vi "Edit PID.vi"(8 "error in (no error)":errorcluster, 11 "Node Ptr":u64 format="%.0x") -> (0 "error out":errorcluster)   [LabVIEW 2015, in "Diagnostics Addon System Explorer.lvlib"]
uses:
  Diagnostics Addon System Explorer.lvlib
  Shared/FG Action.ctl
  Shared/Get Signals from DIDPID.vi
  Shared/Signal Parameters FG.vi
  Shared/GUID Lookup.vi
  <vilib>/NI Veristand/Custom Device API/NI VeriStand - Set Item Property.vi
  <vilib>/NI Veristand/Custom Device API/Set Item Property (U32).vi
  <vilib>/NI Veristand/Custom Device API/NI VeriStand - Get Item Property.vi
  <vilib>/NI Veristand/Custom Device API/Get Item Property (U32).vi
  <vilib>/NI Veristand/Custom Device API/Set Item Property (Double).vi
  <vilib>/NI Veristand/Custom Device API/Set Item Property (String).vi
  <vilib>/NI Veristand/Custom Device API/Get Item Property (Double).vi
  <vilib>/NI Veristand/Custom Device API/Get Item Property (String).vi
  <vilib>/NI Veristand/Custom Device API/NI VeriStand - Get Item Description.vi
  <vilib>/NI Veristand/Custom Device API/NI VeriStand - Get Custom Device Channel Data.vi
  <vilib>/NI Veristand/Custom Device API/Custom Device API.lvlib
  Shared/Diagnostics Addon Shared.lvlib
  <vilib>/NI Veristand/Custom Device Tools/Custom Device Utility Library/Custom Device Utility Library.lvlib
panel:
  in  "Tag":string
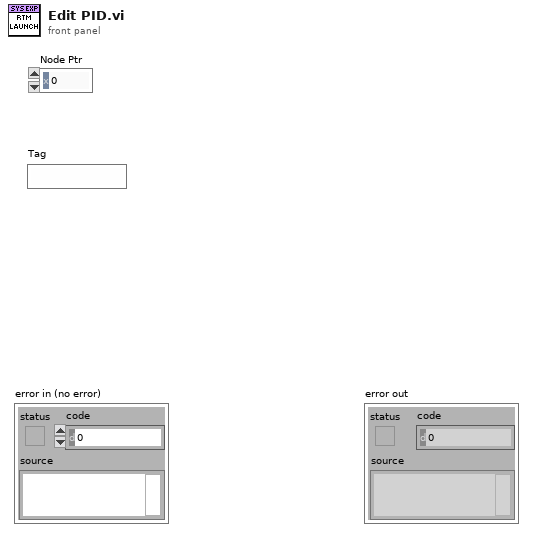
[diagram p1: front panel]
types:
  T1 = typedef "Diagnostics Addon Shared.lvlib/DIDPID Parameters.ctl" = cluster{"Name":string, "Description":string, "ID":u16, "Signals":T2[]}
  T2 = typedef "Diagnostics Addon Shared.lvlib/DIDPID Signal Parameters.ctl" = cluster{"Start Bit":u8, "Length":u8, "Scaling Factor":dbl, "Scaling Offset":dbl, "Minimum":dbl, "Maximum":dbl, "Data Type":u32, "Byte Order":u32, "Default Value":dbl, "Name":string, "Units":string, "Description":string}
  T3 = typedef "Custom Device API.lvlib/Custom Device Item Ref.ctl" = u64
  T4 = typedef "Custom Device API.lvlib/Custom Device Item Info.ctl" = cluster{"Name":string, "Is Channel":bool, "GUID":string, "Is Waveform":bool}
  T5 = typedef "Diagnostics Addon Shared.lvlib/FG Action.ctl" = enum16{"Get", "Set"}
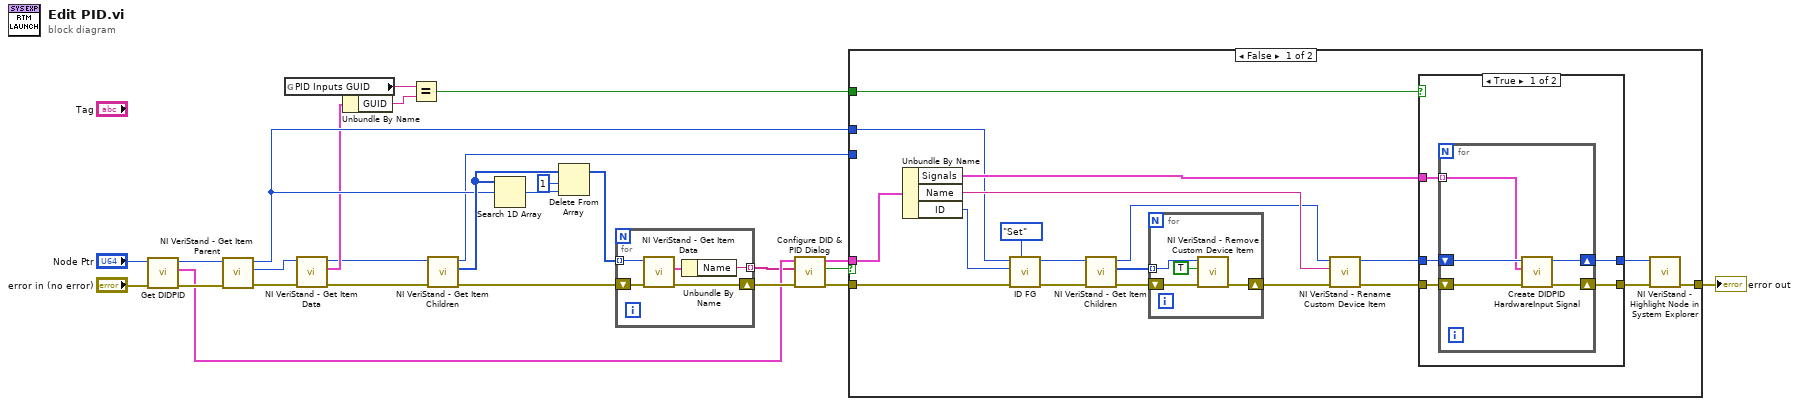
[diagram p0: block diagram]
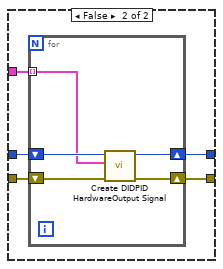
[diagram p2: hidden frame]
diagram:
  n1 = call "Get DIDPID.vi"("error in (no error)"="error in (no error)", "Item Ref in"="Node Ptr") -> ("error out"=w16:errorcluster, "PID In"=w13:T1, "Item Ref out"=w14:T3)  [unwired: 7 in]
  n2 = call <vilib>:"NI VeriStand - Get Item Parent.vi"("error in (no error)"=w16, "Item Ref in"=w14) -> ("error out"=w5:errorcluster, "Parent Ref"=w4:T3, "Item Ref out"=w11:T3)  [unwired: 6 in, 1 out]
  n3 = global read "GUID Lookup.vi" "PID Inputs GUID"() -> (w7:string)
  n4 = call <vilib>:"NI VeriStand - Get Item Data.vi"("error in (no error)"=w5, "Item Ref in"=w4) -> ("error out"=w2:errorcluster, "Item Info"=w8:T4, "Item Ref out"=w3:T3)  [unwired: 6 in, 1 out]
  n5 = Unbundle By Name(w8) -> ("GUID"=w6:string)
  n6 = Equal?(x=w7, y=w6) -> (x = y?=w1:bool)
  n7 = call <vilib>:"NI VeriStand - Get Item Children.vi"("error in (no error)"=w2, "Item Ref in"=w3) -> ("error out"=w26:errorcluster, "Child Refs"=w25:T3[], "Item Ref out"=w10:T3)  [unwired: 6 in, 1 out]
  n8 = Search 1D Array(1D array=w25, element=w11) -> (index of element=w23:i32)  [unwired: 1 in]
  n9 = Delete From Array(array=w25, length=1, index=w23) -> (array with subset deleted=w24:T3[])  [unwired: 1 out]
  n10 = for {
    tunnel: [w29] -> w12 mode=indexing
    shift-right: [w28] -> w18
    shift-left: w26 -> [w30]
    tunnel: w24 -> [w27] mode=indexing
    n11 = call <vilib>:"NI VeriStand - Get Item Data.vi"("error in (no error)"=w30, "Item Ref in"=w27) -> ("error out"=w28:errorcluster, "Item Info"=w31:T4)  [unwired: 8 out]
    n12 = Unbundle By Name(w31) -> ("Name"=w29:string)
  }
  n13 = call "Configure DID & PID Dialog.vi"("error in (no error)"=w18, "Existing PIDs"=w12, "Parameters In"=w13) -> ("error out"=w20:errorcluster, "Cancel PID?"=w19:bool, "Parameters Out"=w21:T1)  [unwired: 6 in]
  n14 = case shown="False" w19 {
    tunnel: w20 -> [w33 w75]
    tunnel: w10 -> [_ _]
    tunnel: w21 -> [w50 _]
    tunnel: [w44 w75] -> w9
    tunnel: w11 -> [w36 _]
    tunnel: w1 -> [w38 _]
    frame False {
      n15 = Unbundle By Name(w50) -> ("Signals"=w41:T2[], "Name"=w49:string, "ID"=w32:u16)
      n16 = call "ID FG.vi"("Action"=FG_Action."Set", "error in (no error)"=w33, "ID"=w32, "Device Item Ref in"=w36) -> ("error out"=w34:errorcluster, "Device Item Ref out"=w35:T3)  [unwired: 5 in, 1 out]
      n17 = call <vilib>:"NI VeriStand - Get Item Children.vi"("error in (no error)"=w34, "Item Ref in"=w35) -> ("error out"=w47:errorcluster, "Child Refs"=w48:T3[], "Item Ref out"=w45:T3)  [unwired: 6 in, 1 out]
      n18 = for {
        tunnel: w48 -> [w74] mode=indexing
        shift-right: [w71] -> w46
        shift-left: w47 -> [w73]
        n19 = call <vilib>:"NI VeriStand - Remove Custom Device Item.vi"("error in (no error)"=w73, "Force Delete (F)"=TRUE, "Item Ref in"=w74) -> ("error out"=w71:errorcluster)  [unwired: 7 in, 1 out]
      }
      n20 = call <vilib>:"NI VeriStand - Rename Custom Device Item.vi"("error in (no error)"=w46, "New Name"=w49, "Item Ref in"=w45) -> ("error out"=w43:errorcluster, "Item Ref out"=w42:T3)  [unwired: 1 in, 6 out]
      n21 = case shown="True" w38 {
        tunnel: w42 -> [w55 w65]
        tunnel: w41 -> [w54 w64]
        tunnel: [w53 w63] -> w40
        tunnel: w43 -> [w52 w62]
        tunnel: [w51 w61] -> w39
        frame True {
          n22 = for {
            shift-right: [w59] -> w53
            shift-left: w52 -> [w60]
            tunnel: w54 -> [w57] mode=indexing
            shift-right: [w56] -> w51
            shift-left: w55 -> [w58]
            n23 = call "Create DIDPID HardwareInput Signal.vi"("error in (no error)"=w60, "Signal Parameters"=w57, "Section Ptr"=w58) -> ("error out"=w59:errorcluster, "Section Ptr out"=w56:T3)  [unwired: 7 in]
          }
        }
        frame False {
          n24 = for {
            shift-right: [w67] -> w63
            shift-left: w62 -> [w69]
            tunnel: w64 -> [w68] mode=indexing
            shift-right: [w66] -> w61
            shift-left: w65 -> [w70]
            n25 = call "Create DIDPID HardwareOutput Signal.vi"("error in (no error)"=w69, "Signal Parameters"=w68, "Section Ptr"=w70) -> ("error out"=w67:errorcluster, "Section Ptr out"=w66:T3)  [unwired: 7 in]
          }
        }
      }
      n26 = call <vilib>:"NI VeriStand - Highlight Node in System Explorer.vi"("error in (no error)"=w40, "Item Ref in"=w39) -> ("error out"=w44:errorcluster)  [unwired: 8 in, 1 out]
    }
    frame True {
    }
  }
  "error out" <- w9
